vi "SubPanel Controls.vi"() -> ()   [LabVIEW 2011, in "Scan Engine Custom Device.lvlib"]
uses:
  Scan Engine Custom Device.lvlib
panel:
  in  "SubPanel Event":string="SubPanel Event"
  in  "error out":string="error out"
  in  "Header":string="Header"
  in  "error in (no error)":string="error in (no error)"
  in  "Node Ptr":string="Node Ptr"
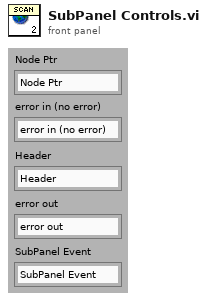
[diagram p1: front panel]
diagram:
